vi "Gone Around.vi"(11 "Impenetrable in":refnum<class "Impenetrable.lvclass">) -> (3 "Impenetrable out":refnum<class "Impenetrable.lvclass">)   [LabVIEW 2015, in "Impenetrable.lvclass"]
uses:
  Impenetrable.lvclass
  Impenetrable.lvclass/Impenetrable.ctl
  SubVIs/Read-Only Globals.vi
  SubVIs/Globals (private).vi
  Globals.vi
  Square/Square.lvclass
panel:
  out "Rain Round":i32
  out "Round":i32
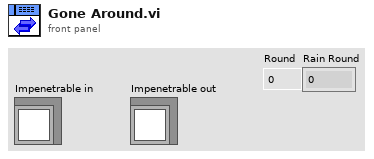
[diagram p1: front panel]
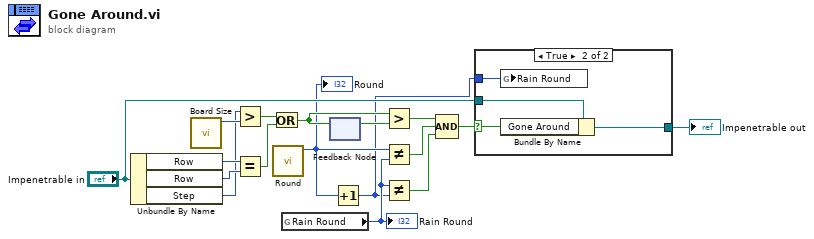
[diagram p0: block diagram]
diagram:
  n1 = Unbundle By Name("Impenetrable in") -> ("Row"=w15:i32, "Row"=w13:i32, "Step"=w11:i32)
  n2 = call "Board Size.vi"() -> ("Board Size"=w12:i32)  [unwired: 11 in]
  n3 = Greater?(x=w11, y=w12) -> (0:w10:bool)
  n4 = Equal?(x=w15, y=w13) -> (x = y?=w14:bool)
  n5 = Or(x=w10, y=w14) -> (x .or. y?=w9:bool)
  n6 = call "Round.vi"() -> ("Round"=w4:i32)  [unwired: 11 in]
  "Round" <- w4
  n7 = global read "Globals.vi" "Rain Round"() -> (w5:i32)
  "Rain Round" <- w5
  n8 = feedback-in #1(w9) -> ()
  n9 = feedback #1() -> (w8:bool)  [unwired: 1 in]
  n10 = Increment(x=w4) -> (x+1=w1:i32)
  n11 = Greater?(x=w9, y=w8) -> (0:w3:bool)
  n12 = Not Equal?(x=w4, y=w5) -> (x != y?=w7:bool)
  n13 = Not Equal?(x=w5, y=w1) -> (x != y?=w6:bool)
  n14 = Compound Arithmetic op=AND(w3, w7, w6) -> (w2:bool)
  n15 = case shown="True" w2 {
    selector: w2 -> [_ w20]
    tunnel: "Impenetrable in" -> [w18 w21]
    tunnel: [w18 w22] -> w17
    tunnel: w1 -> [_ w19]
    frame False {
    }
    frame True {
      n16 = global write "Globals.vi" "Rain Round"(w19) -> ()
      n17 = Bundle By Name(cluster=w21, "Gone Around"=w20) -> (w22:refnum<class "Impenetrable.lvclass">)
    }
  }
  "Impenetrable out" <- w17
